vi "Test40 DCIR.vi"(7 "3P4S":bool, 8 "errin":errorcluster, 10 "SN":string="0B5MEVA000CA1JC1M0000041", 11 "L2T 2":T2 caption="Limites de test pris en compte") -> (0 "errout":errorcluster, 1 "Out":T3, 2 "cluster de sortie":T4, 3 "v1":string, 4 "test OK?":bool, 5 "RDCIR":dbl)   [LabVIEW 2020]
uses:
  Ctrl/L2T.ctl
  <userlib>/PCAN Basic/Controls/Channel.ctl
  <userlib>/PCAN Basic/Controls/BaudrateEenum.ctl
  0bef8869-a7f7-460e-a649-f0efb8154831.vi
  VarGLO/Global PEAK.vi
  02 SLIM ZEN WS 500/SubVi/VG_progressBar.vi
  <userlib>/Alex_Peak_lib/PEAK_lib_ALEX.lvlib
  <userlib>/PCAN Basic/PCANBasic.lvlib
  <instrlib>/IT6000C/IT6000C.lvlib
panel:
  out "chaîne concaténée":string
  out "errout 2":errorcluster caption="errout"
  out "T40":T1=enum."PCAN_USBBUS1"
  in  "stop":bool
  # "Pre DCIR_____________________________________"
  # "intra DCIR_____________________________________"
  # "Post DCIR_____________________________________"
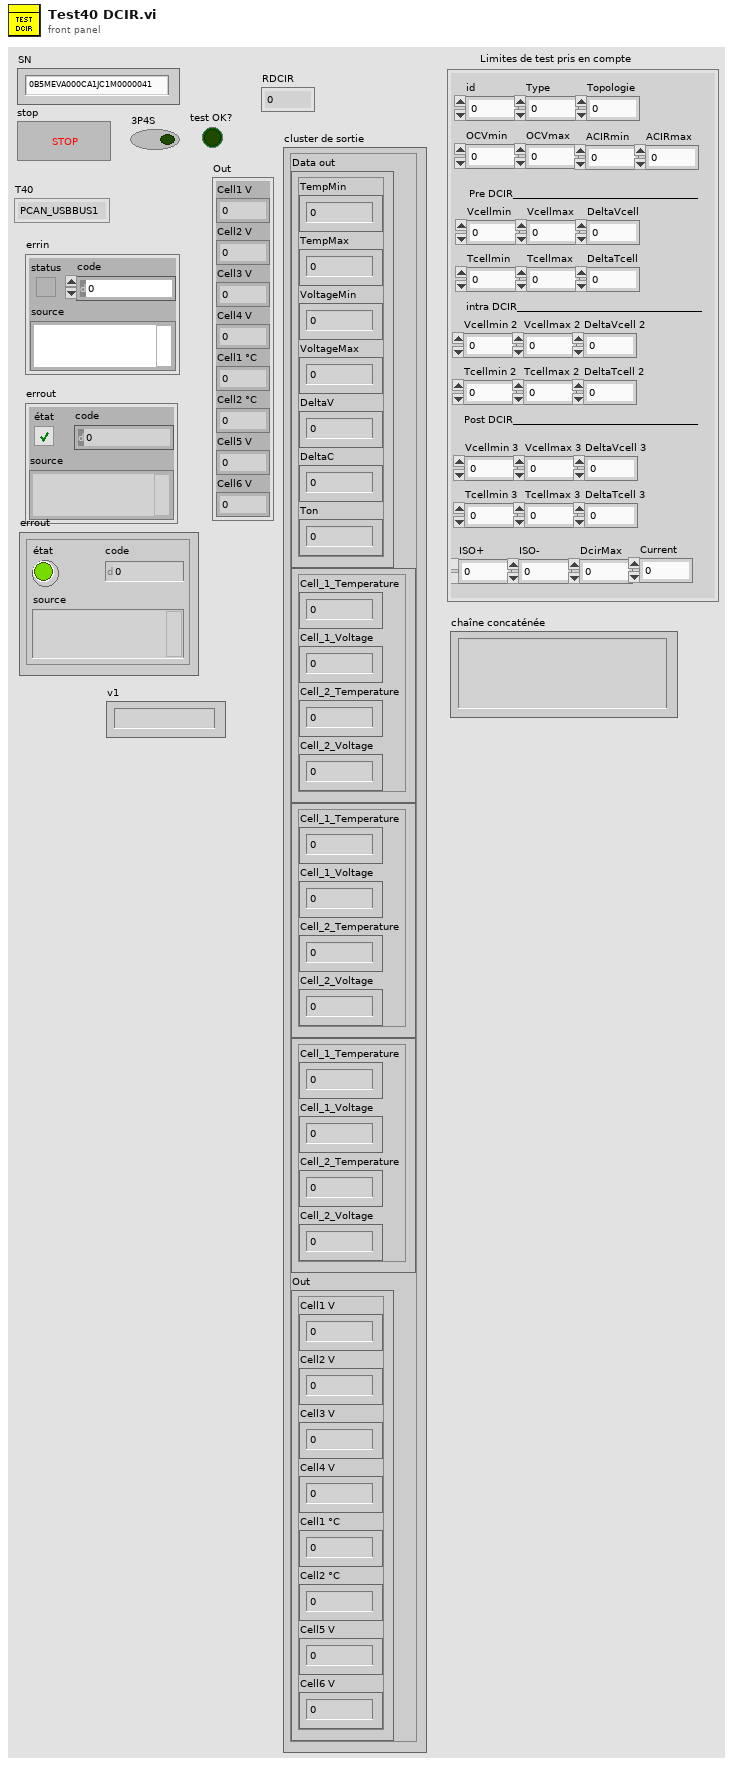
[diagram p1: front panel]
types:
  T1 = typedef "PCANBasic.lvlib/Channel.ctl" = enum16{"PCAN_NONEBUS", "not used1", "not used2", "not used3", "not used4", "not used5", "not used6", "not used7", "not used8", "not used9", "not used10", "not used11", "not used12", "not used13", "not used14", "not used15", "not used16", "not used17", "not used18", "not used19", "not used20", "not used21", "not used22", "not used23", "not used24", "not used25", "not used26", "not used27", "not used28", "not used29", "not used30", "not used31", "not used32", "PCAN_ISABUS1", "PCAN_ISABUS2", "PCAN_ISABUS3", "PCAN_ISABUS4", "PCAN_ISABUS5", "PCAN_ISABUS6", "PCAN_ISABUS7", "PCAN_ISABUS8", "not used41", "not used42", "not used43", "not used44", "not used45", "not used46", "not used47", "not used48", "PCAN_DNGBUS1", "not used50", "not used51", "not used52", "not used53", "not used54", "not used55", "not used56", "not used57", "not used58", "not used59", "not used60", "not used61", "not used62", "not used63", "not used64", "PCAN_PCIBUS1", "PCAN_PCIBUS2", "PCAN_PCIBUS3", "PCAN_PCIBUS4", "PCAN_PCIBUS5", "PCAN_PCIBUS6", "PCAN_PCIBUS7", "PCAN_PCIBUS8", "not used73", "not used74", "not used75", "not used76", "not used77", "not used78", "not used79", "not used80", "PCAN_USBBUS1", "PCAN_USBBUS2", "PCAN_USBBUS3", "PCAN_USBBUS4", "PCAN_USBBUS5", "PCAN_USBBUS6", "PCAN_USBBUS7", "PCAN_USBBUS8", "Not used89", "Not used90", "Not used91", "Not used92", "Not used93", "Not used94", "Not used95", "Not used96", "PCAN_PCCBUS1", "PCAN_PCCBUS2"}
  T2 = typedef "L2T.ctl" = cluster{"id":dbl, "Type":dbl, "OCVmin":dbl, "OCVmax":dbl, "ACIRmin":dbl, "ACIRmax":dbl, "Vcellmin":dbl, "Vcellmax":dbl, "DeltaVcell":dbl, "Tcellmin":dbl, "Tcellmax":dbl, "DeltaTcell":dbl, "ISO+":dbl, "ISO-":dbl, "DcirMax":dbl, "Current":dbl, "Topologie":dbl, "Vcellmin 2":dbl, "Vcellmax 2":dbl, "DeltaVcell 2":dbl, "Tcellmin 2":dbl, "Tcellmax 2":dbl, "DeltaTcell 2":dbl, "Vcellmin 3":dbl, "Vcellmax 3":dbl, "DeltaVcell 3":dbl, "Tcellmin 3":dbl, "Tcellmax 3":dbl, "DeltaTcell 3":dbl}
  T3 = cluster{"Cell1 V":sgl, "Cell2 V":sgl, "Cell3 V":sgl, "Cell4 V":sgl, "Cell1 °C":sgl, "Cell2 °C":sgl, "Cell5 V":sgl, "Cell6 V":sgl}
  T4 = cluster{"Data out":cluster{"TempMin":sgl, "TempMax":sgl, "VoltageMin":sgl, "VoltageMax":sgl, "DeltaV":sgl, "DeltaC":sgl, "Ton":sgl}, "Cluster":cluster{"Cell_1_Temperature":sgl, "Cell_1_Voltage":sgl, "Cell_2_Temperature":sgl, "Cell_2_Voltage":sgl}, "Cluster":cluster{"Cell_1_Temperature":sgl, "Cell_1_Voltage":sgl, "Cell_2_Temperature":sgl, "Cell_2_Voltage":sgl}, "Cluster":cluster{"Cell_1_Temperature":sgl, "Cell_1_Voltage":sgl, "Cell_2_Temperature":sgl, "Cell_2_Voltage":sgl}, "Out":cluster{"Cell1 V":sgl, "Cell2 V":sgl, "Cell3 V":sgl, "Cell4 V":sgl, "Cell1 °C":sgl, "Cell2 °C":sgl, "Cell5 V":sgl, "Cell6 V":sgl}}
  T5 = typedef "PCANBasic.lvlib/BaudrateEenum.ctl" = enum16{"CAN_Baud_1M", "CAN_Baud_800K", "CAN_BAUD_500K", "CAN_BAUD_250K", "CAN_BAUD_125K", "CAN_BAUD_100K", "CAN_BAUD_95K", "CAN_BAUD_83K", "CAN_BAUD_50K", "CAN_BAUD_47K", "CAN_BAUD_33K", "CAN_BAUD_20K", "CAN_BAUD_10K", "CAN_BAUD_5K", "User Baudrate"}
  T6 = cluster{"TempMin":sgl, "TempMax":sgl, "VoltageMin":sgl, "VoltageMax":sgl, "DeltaV":sgl, "DeltaC":sgl, "Ton":sgl}
  T7 = cluster{"Cell_1_Temperature":sgl, "Cell_1_Voltage":sgl, "Cell_2_Temperature":sgl, "Cell_2_Voltage":sgl}
  T8 = cluster{"ID":u32, "MSGTYPE":u8, "LEN":u8, "DATA[0]":u8, "DATA[1]":u8, "DATA[2]":u8, "DATA[3]":u8, "DATA[4]":u8, "DATA[5]":u8, "DATA[6]":u8, "DATA[7]":u8}
  T9 = cluster{"Data out":cluster{"TempMin":sgl, "TempMax":sgl, "VoltageMin":sgl, "VoltageMax":sgl, "DeltaV":sgl, "DeltaC":sgl, "Ton":sgl}, cluster{"Cell_1_Temperature":sgl, "Cell_1_Voltage":sgl, "Cell_2_Temperature":sgl, "Cell_2_Voltage":sgl}, cluster{"Cell_1_Temperature":sgl, "Cell_1_Voltage":sgl, "Cell_2_Temperature":sgl, "Cell_2_Voltage":sgl}, cluster{"Cell_1_Temperature":sgl, "Cell_1_Voltage":sgl, "Cell_2_Temperature":sgl, "Cell_2_Voltage":sgl}, "Out":cluster{"Cell1 V":sgl, "Cell2 V":sgl, "Cell3 V":sgl, "Cell4 V":sgl, "Cell1 °C":sgl, "Cell2 °C":sgl, "Cell5 V":sgl, "Cell6 V":sgl}}
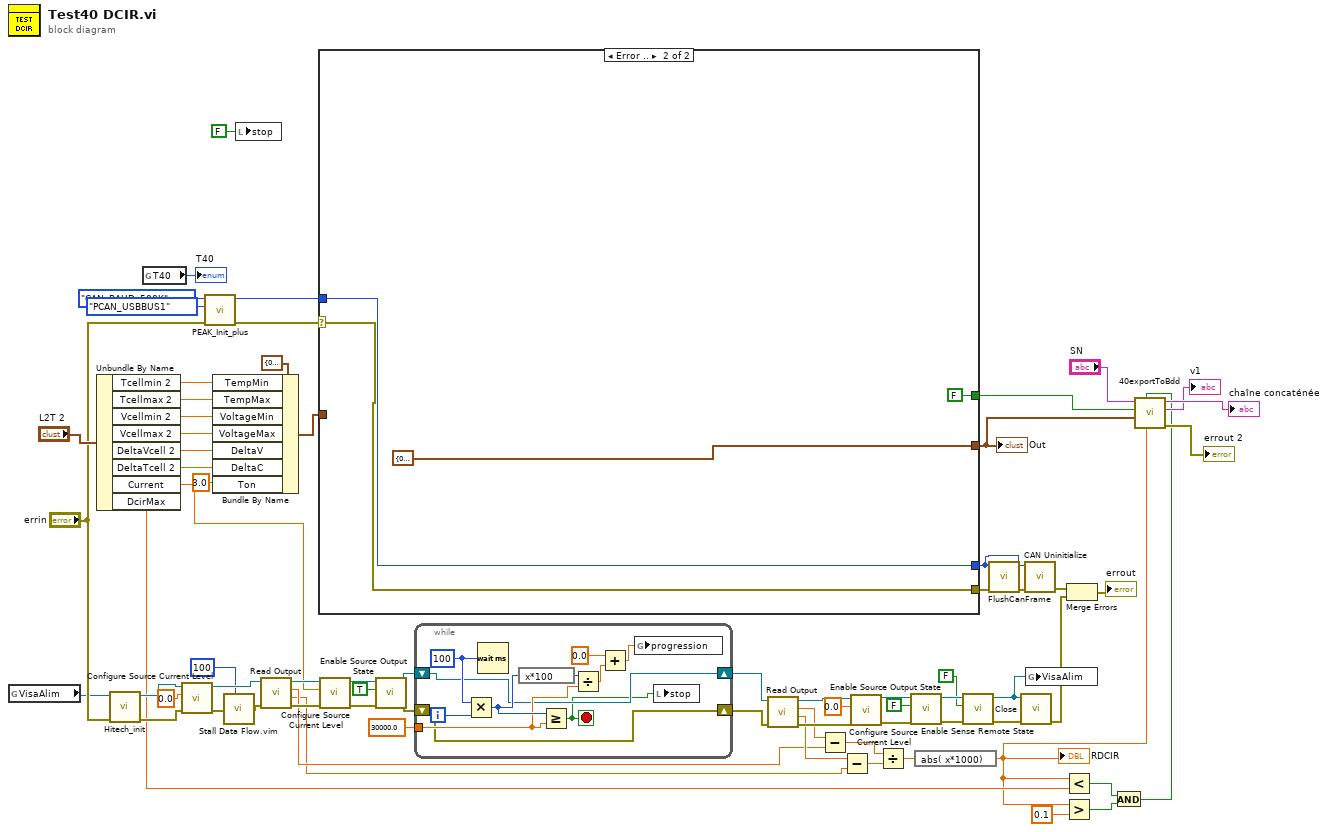
[diagram p0: block diagram]
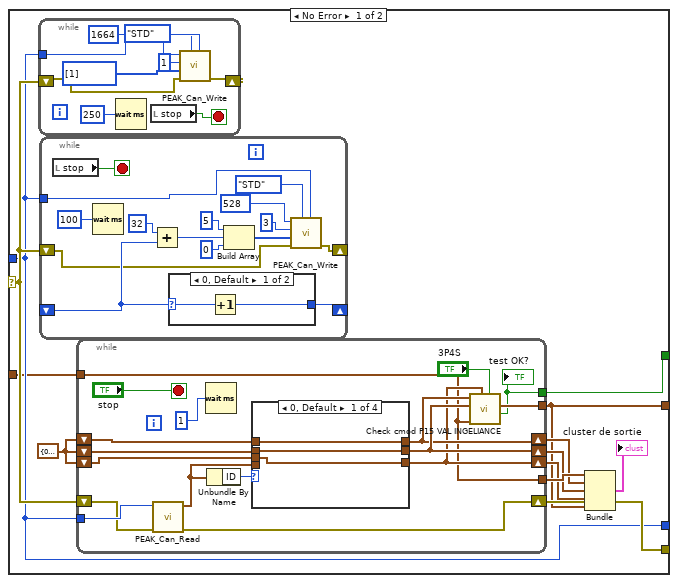
[diagram p2: hidden frame]
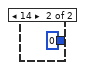
[diagram p3: hidden frame]
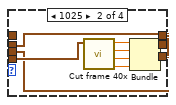
[diagram p4: hidden frame]
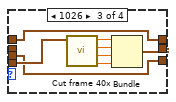
[diagram p5: hidden frame]
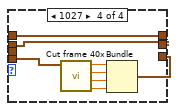
[diagram p6: hidden frame]
diagram:
  n1 = global read "Global PEAK.vi" "VisaAlim"() -> (w20:refnum<visa-resource-name>)
  n2 = Unbundle By Name("L2T 2") -> ("Tcellmin 2"=w67:dbl, "Tcellmax 2"=w66:dbl, "Vcellmin 2"=w65:dbl, "Vcellmax 2"=w64:dbl, "DeltaVcell 2"=w63:dbl, "DeltaTcell 2"=w62:dbl, "Current"=w29:dbl, "DcirMax"=w14:dbl)
  n3 = call "Hitech_init.vi"("errin"="errin", "VISA HITECH"=w20) -> ("error out"=w22:errorcluster, "VisaHitech"=w19:refnum<visa-resource-name>)  [unwired: 8 in]
  n4 = global read "Global PEAK.vi" "T40"() -> (→"T40":T1)
  n5 = call <instrlib>:"Configure Source Current Level.vi"("error in (no error)"=w22, "Value(0)"=0.0, "VISA resource name"=w19) -> ("error out"=w25:errorcluster, "VISA resource name out"=w57:refnum<visa-resource-name>)  [unwired: 7 in]
  n6 = call "PEAK_Init_plus.vi"("errin"="errin", "Channel"=Channel."PCAN_USBBUS1", "BTR0BTR1"=BaudrateEenum."CAN_BAUD_500K") -> ("errout"=w71:errorcluster, "Channel out"=w72:T1)  [unwired: 7 in]
  n7 = Bundle By Name(cluster=T6 {"TempMin"=0.0, "TempMax"=0.0, "VoltageMin"=0.0, "VoltageMax"=0.0, "DeltaV"=0.0, "DeltaC"=0.0, "Ton"=0.0} ("Data out"), "TempMin"=w67, "TempMax"=w66, "VoltageMin"=w65, "VoltageMax"=w64, "DeltaV"=w63, "DeltaC"=w62, "Ton"=sgl 3.0) -> (w60:T6)
  n8 = call "Stall Data Flow.vim"("value in"=w25, "milliseconds to wait"=u32 100) -> ("value out"=w24:errorcluster)  [unwired: 1 out]
  n9 = local write "stop"(FALSE ("stop")) -> ()
  n10 = call <instrlib>:"Read Output.vi"("error in (no error)"=w24, "VISA resource name"=w57) -> ("error out"=w56:errorcluster, "Actual Current Level (A)"=w34:dbl, "Actual Voltage Level (V)"=w35:dbl, "VISA resource name out"=w55:refnum<visa-resource-name>)  [unwired: 6 in]
  n11 = case shown="Error .." w71 {
    selector: w71 -> [w84 w159]
    tunnel: w72 -> [w82 w158]
    tunnel: [w83 w159] -> w70
    tunnel: [w82 w158] -> w28
    tunnel: w60 -> [w81 _]
    tunnel: [w74 T3 {"Cell1 V"=0.0, "Cell2 V"=0.0, "Cell3 V"=0.0, "Cell4 V"=0.0, "Cell1 °C"=0.0, "Cell2 °C"=0.0, "Cell5 V"=0.0, "Cell6 V"=0.0} ("Out")] -> w15
    tunnel: [w73 FALSE ("ok global")] -> w1
    frame No Error {
      w80 = T7 {"Cell_1_Temperature"=0.0, "Cell_1_Voltage"=0.0, "Cell_2_Temperature"=0.0, "Cell_2_Voltage"=0.0}
      n12 = while {
        tunnel: w82 -> [w89]
        shift-right: [w91] -> _
        shift-left: w84 -> [w86]
        stop <- w85 stop-if-true
        n13 = Wait (ms)(milliseconds to wait=u32 250 ("attente (ms)")) -> ()  [unwired: 1 out]
        n14 = local read "stop"() -> (w85:bool)
        n15 = call <userlib>:"PEAK_Can_Write.vi"("CAN Handle"=w89, "MSG type"=enum8{"STD", "RTR", "XTD", "XTD RTR", "STATUS"}."STD", "errin"=w86, "CAN Data"=u8[] [1], "DLC (8)"=u8 1, "Identifier"=u32 1664) -> ("errout"=w91:errorcluster)  [unwired: 5 in]
      }
      n16 = while {
        tunnel: w82 -> [w96]
        shift-right: [w108] -> _
        shift-left: _ -> [w107]
        shift-right: [w106] -> _
        shift-left: w84 -> [w94]
        stop <- w95 stop-if-true
        n17 = local read "stop"() -> (w95:bool)
        n18 = Wait (ms)(milliseconds to wait=u32 100 ("attente (ms)")) -> ()  [unwired: 1 out]
        n19 = Add(x=u8 32, y=w107) -> (x+y=w101:i32)
        n20 = case shown="0, Default" w107 {
          selector: w107 -> [w110 _]
          tunnel: [w109 0] -> w108
          frame 0, Default {
            n21 = Increment(x=w110) -> (x+1=w109:i32)
          }
          frame 14 {
          }
        }
        n22 = Build Array(u8 5 ("élément"), w101, u8 0 ("élément")) -> (w100:i32[])
        n23 = call <userlib>:"PEAK_Can_Write.vi"("CAN Handle"=w96, "MSG type"=enum8{"STD", "RTR", "XTD", "XTD RTR", "STATUS"}."STD", "errin"=w94, "CAN Data"=w100, "DLC (8)"=u8 3, "Identifier"=u32 528) -> ("errout"=w106:errorcluster)  [unwired: 5 in]
      }
      n24 = while {
        shift-right: [w122] -> w83
        shift-left: w84 -> [w126]
        shift-right: [w120] -> w78
        shift-left: w80 -> [w124]
        shift-right: [w121] -> w77
        shift-left: w80 -> [w123]
        tunnel: w82 -> [w127]
        tunnel: [w119] -> w74
        tunnel: w81 -> [w114]
        shift-right: [w116] -> w76
        shift-left: w80 -> [w118]
        tunnel: [w114] -> w79
        tunnel: [w112] -> w73
        stop <- "stop" stop-if-true
        n25 = call <userlib>:"PEAK_Can_Read.vi"("errin"=w126, "Channel out"=w127) -> ("errout"=w122:errorcluster, "MessageBuffer out"=w125:T8)  [unwired: 7 in, 1 out]
        n26 = Wait (ms)(milliseconds to wait=u32 1 ("attente (ms)")) -> ()  [unwired: 1 out]
        n27 = Unbundle By Name(w125) -> ("ID"=w117:u32)
        n28 = case shown="0, Default" w117 {
          tunnel: w125 -> [_ w134 w142 w151]
          tunnel: [w131 w135 w141 w149] -> w120
          tunnel: [w130 w133 w143 w148] -> w121
          tunnel: w124 -> [w131 _ w141 w149]
          tunnel: w123 -> [w130 w133 _ w148]
          tunnel: [w129 w132 w140 w150] -> w116
          tunnel: w118 -> [w129 w132 w140 _]
          frame 0, Default {
          }
          frame 1025 {
            n29 = call "Cut frame 40x.vi"("MessageBuffer out"=w134) -> ("Cell_2_Voltage"=w136:sgl, "Cell_2_Temperature"=w137:sgl, "Cell_1_Voltage"=w138:sgl, "Cell_1_Temperature"=w139:sgl)  [unwired: 7 in]
            n30 = Bundle("Cell_1_Temperature"=w139, "Cell_1_Voltage"=w138, "Cell_2_Temperature"=w137, "Cell_2_Voltage"=w136) -> (w135:T7)  [unwired: 1 in]
          }
          frame 1026 {
            n31 = call "Cut frame 40x.vi"("MessageBuffer out"=w142) -> ("Cell_2_Voltage"=w144:sgl, "Cell_2_Temperature"=w145:sgl, "Cell_1_Voltage"=w146:sgl, "Cell_1_Temperature"=w147:sgl)  [unwired: 7 in]
            n32 = Bundle("Cell_1_Temperature"=w147, "Cell_1_Voltage"=w146, "Cell_2_Temperature"=w145, "Cell_2_Voltage"=w144) -> (w143:T7)  [unwired: 1 in]
          }
          frame 1027 {
            n33 = call "Cut frame 40x.vi"("MessageBuffer out"=w151) -> ("Cell_2_Voltage"=w152:sgl, "Cell_2_Temperature"=w153:sgl, "Cell_1_Voltage"=w154:sgl, "Cell_1_Temperature"=w155:sgl)  [unwired: 7 in]
            n34 = Bundle("Cell_1_Temperature"=w155, "Cell_1_Voltage"=w154, "Cell_2_Temperature"=w153, "Cell_2_Voltage"=w152) -> (w150:T7)  [unwired: 1 in]
          }
        }
        n35 = call "Check cmod P15 VAL INGELIANCE.vi"("3P4S"="3P4S", "Cell 5 et 6"=w116, "Limites"=w114, "Cell 3 et 4"=w121, "Cell 1 et 2"=w120) -> ("ok global"=w112:bool, "Out"=w119:T3)  [unwired: 2 in, 3 out]
        "test OK?" <- w112
      }
      n36 = Bundle("Data out"=w79, w78, w77, w76, "Out"=w74) -> (→"cluster de sortie":T9)  [unwired: 1 in]
    }
    frame Error {
    }
  }
  "Out" <- w15
  n37 = call <instrlib>:"Configure Source Current Level.vi"("error in (no error)"=w56, "Value(0)"=w29, "VISA resource name"=w55) -> ("error out"=w54:errorcluster, "VISA resource name out"=w53:refnum<visa-resource-name>)  [unwired: 7 in]
  n38 = call <instrlib>:"Enable Source Output State.vi"("error in (no error)"=w54, "Enable(True)"=TRUE, "VISA resource name"=w53) -> ("error out"=w49:errorcluster, "VISA resource name out"=w50:refnum<visa-resource-name>)  [unwired: 7 in]
  n39 = while {
    tunnel: sgl 30000.0 ("Ton") -> [w166]
    shift-right: [w164] -> w36
    shift-left: w50 -> [w164]
    shift-right: [w165] -> w37
    shift-left: w49 -> [w165]
    i -> [w170]
    stop <- w160 stop-if-true
    w169 = u32 100 ("attente (ms)")
    n40 = Multiply(x=w169, y=w170) -> (x*y=w167:u32)
    n41 = Wait (ms)(milliseconds to wait=w169) -> ()  [unwired: 1 out]
    n42 = expression code="x*100"(w167) -> (w168:u32)
    n43 = Greater Or Equal?(x=w167, y=w166) -> (x >= y?=w160:bool)
    n44 = Divide(x=w168, y=w166) -> (x/y=w163:sgl)
    n45 = Add(x=sgl 0.0, y=w163) -> (x+y=w162:sgl)
    n46 = global write "VG_progressBar.vi" "progression"(w162) -> ()
    n47 = local write "stop"(w160) -> ()
  }
  n48 = call <instrlib>:"Read Output.vi"("error in (no error)"=w37, "VISA resource name"=w36) -> ("error out"=w47:errorcluster, "Actual Current Level (A)"=w39:dbl, "Actual Voltage Level (V)"=w40:dbl, "VISA resource name out"=w46:refnum<visa-resource-name>)  [unwired: 6 in]
  n49 = Subtract(x=w40, y=w35) -> (x-y=w38:dbl)
  n50 = Subtract(x=w39, y=w34) -> (x-y=w42:dbl)
  n51 = call <instrlib>:"Configure Source Current Level.vi"("error in (no error)"=w47, "Value(0)"=0.0, "VISA resource name"=w46) -> ("error out"=w45:errorcluster, "VISA resource name out"=w44:refnum<visa-resource-name>)  [unwired: 7 in]
  n52 = Divide(x=w38, y=w42) -> (x/y=w41:dbl)
  n53 = call <instrlib>:"Enable Source Output State.vi"("error in (no error)"=w45, "Enable(True)"=FALSE, "VISA resource name"=w44) -> ("error out"=w4:errorcluster, "VISA resource name out"=w6:refnum<visa-resource-name>)  [unwired: 7 in]
  n54 = expression code="abs( x*1000)"(w41) -> (w11:dbl)
  "RDCIR" <- w11
  n55 = call <instrlib>:"Enable Sense Remote State.vi"("error in (no error)"=w4, "Enable(True)"=FALSE, "VISA resource name"=w6) -> ("error out"=w3:errorcluster, "VISA resource name out"=w5:refnum<visa-resource-name>)  [unwired: 7 in]
  n56 = call <userlib>:"FlushCanFrame.vi"("errin"=w70, "Channel in"=w28) -> ("error out"=w69:errorcluster)  [unwired: 9 in]
  n57 = call <instrlib>:"Close.vi"("error in (no error)"=w3, "VISA resource name"=w5) -> ("error out"=w18:errorcluster)  [unwired: 9 in]
  n58 = call <userlib>:"CAN Uninitialize.vi"("error in (no error)"=w69, "Channel"=w28) -> ("error out"=w32:errorcluster)  [unwired: 7 in, 2 out]
  n59 = global write "Global PEAK.vi" "VisaAlim"(w5) -> ()
  n60 = Less?(x=w11, y=w14) -> (x < y?=w8:bool)
  n61 = Greater?(x=w11, y=0.1) -> (0:w9:bool)
  n62 = Merge Errors(w32, w18) -> (→"errout":errorcluster)
  n63 = And(x=w8, y=w9) -> (x .and. y?=w7:bool)
  n64 = call "40exportToBdd.vi"("Dcir"=w11, "dcirOK?"=w7, "Datain"=w15, "test OK?"=w1, "SN"="SN") -> ("error out"=→"errout 2":errorcluster, "PLC requet"=→"v1":string, "chaîne concaténée"=→"chaîne concaténée":string)  [unwired: 4 in]
